vi "DPT RMC Range Calculation.vi"(8 "Error In":errorcluster, 11 "Dryer IMC Data Input":T1={"Measured IMC (lbs)"=7.0, "Actual Initial RMC (%)"=7.0, "RMC (Desired %)"=100.0, "Bone Dry Wt(lbs)"=7.0, "Tolerance(%)"=5.0, "Actual Final RMC (%)"=7.0, "CEF (lbf/kWh)"=0.0, "Minimum Weight (lbf)"=0.0, "Average Weight (lbf)"=0.0, "Maximum Weight (lbf)"=0.0, "Measured IMC In Range?"=FALSE, "Moisture Reduction Factor"=55.5, "Field Use Factor"=1.04, "Empty Dryer Cold Weigth"=0.0, "Energy Standard"=enum."D2-Automatic Dryer", "Weight Cloth (lbs)"=0.0, "Relative Moisture Content (%)"=0.0, "Relative Moisture Content - Avg (%)"=0.0} {"Maximum Weight (lbf)" format="%03_6g"; "Average Weight (lbf)" format="%03_6g"; "Minimum Weight (lbf)" format="%03_6g"; "CEF (lbf/kWh)" format="%03_6g"; "Actual Final RMC (%)" format="%03_6g"; "Tolerance(%)" format="%0#_6g"; "Bone Dry Wt(lbs)" format="%03_6g"; "RMC (Desired %)" format="%0#_6g"; "Actual Initial RMC (%)" format="%03_6g"; "Measured IMC (lbs)" format="%0#_6g"}) -> (0 "Error Out":errorcluster, 3 "Dryer IMC Data Output":T1={"Measured IMC (lbs)"=7.0, "Actual Initial RMC (%)"=7.0, "RMC (Desired %)"=100.0, "Bone Dry Wt(lbs)"=7.0, "Tolerance(%)"=5.0, "Actual Final RMC (%)"=7.0, "CEF (lbf/kWh)"=0.0, "Minimum Weight (lbf)"=0.0, "Average Weight (lbf)"=0.0, "Maximum Weight (lbf)"=0.0, "Measured IMC In Range?"=FALSE, "Moisture Reduction Factor"=55.5, "Field Use Factor"=1.04, "Empty Dryer Cold Weigth"=0.0, "Energy Standard"=enum."D2-Automatic Dryer", "Weight Cloth (lbs)"=0.0, "Relative Moisture Content (%)"=0.0, "Relative Moisture Content - Avg (%)"=0.0} {"Maximum Weight (lbf)" format="%03_6g"; "Average Weight (lbf)" format="%03_6g"; "Minimum Weight (lbf)" format="%03_6g"; "CEF (lbf/kWh)" format="%03_6g"; "Actual Final RMC (%)" format="%03_6g"; "Tolerance(%)" format="%0#_6g"; "Bone Dry Wt(lbs)" format="%03_6g"; "RMC (Desired %)" format="%0#_6g"; "Actual Initial RMC (%)" format="%03_6g"; "Measured IMC (lbs)" format="%0#_6g"})   [LabVIEW 2020, in "File Setup.lvlib"]
uses:
  File Setup.lvlib
  Type Definition/DPT IMC Data.ctl
  Washer DOE/Type Definitions/DOE Dryer Standard.ctl
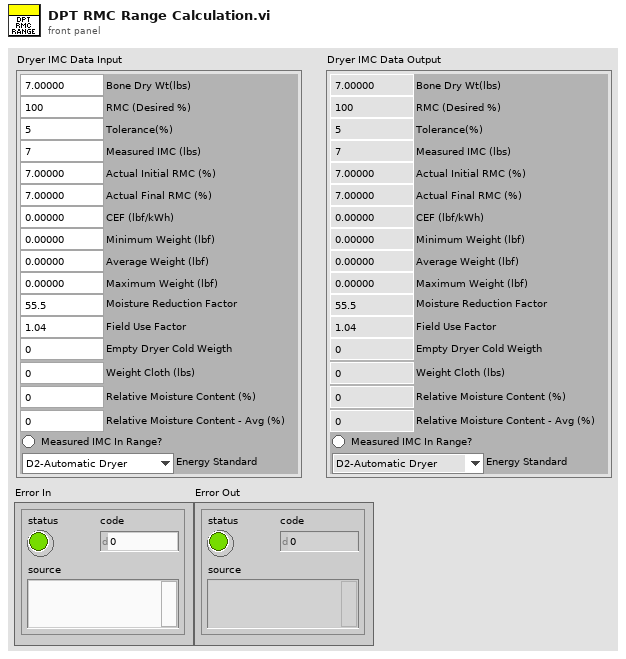
[diagram p1: front panel]
types:
  T1 = typedef "DPT IMC Data.ctl" = cluster{"Measured IMC (lbs)":dbl, "Actual Initial RMC (%)":dbl, "RMC (Desired %)":dbl, "Bone Dry Wt(lbs)":dbl, "Tolerance(%)":dbl, "Actual Final RMC (%)":dbl, "CEF (lbf/kWh)":dbl, "Minimum Weight (lbf)":dbl, "Average Weight (lbf)":dbl, "Maximum Weight (lbf)":dbl, "Measured IMC In Range?":bool, "Moisture Reduction Factor":dbl, "Field Use Factor":dbl, "Empty Dryer Cold Weigth":dbl, "Energy Standard":T2, "Weight Cloth (lbs)":dbl, "Relative Moisture Content (%)":dbl, "Relative Moisture Content - Avg (%)":dbl}
  T2 = typedef "DOE Dryer Standard.ctl" = enum16{"D2-Automatic Dryer", "D2-Timer Dryer", "D1-Automatic Dryer", "D1-Timer Dryer", "Other"}
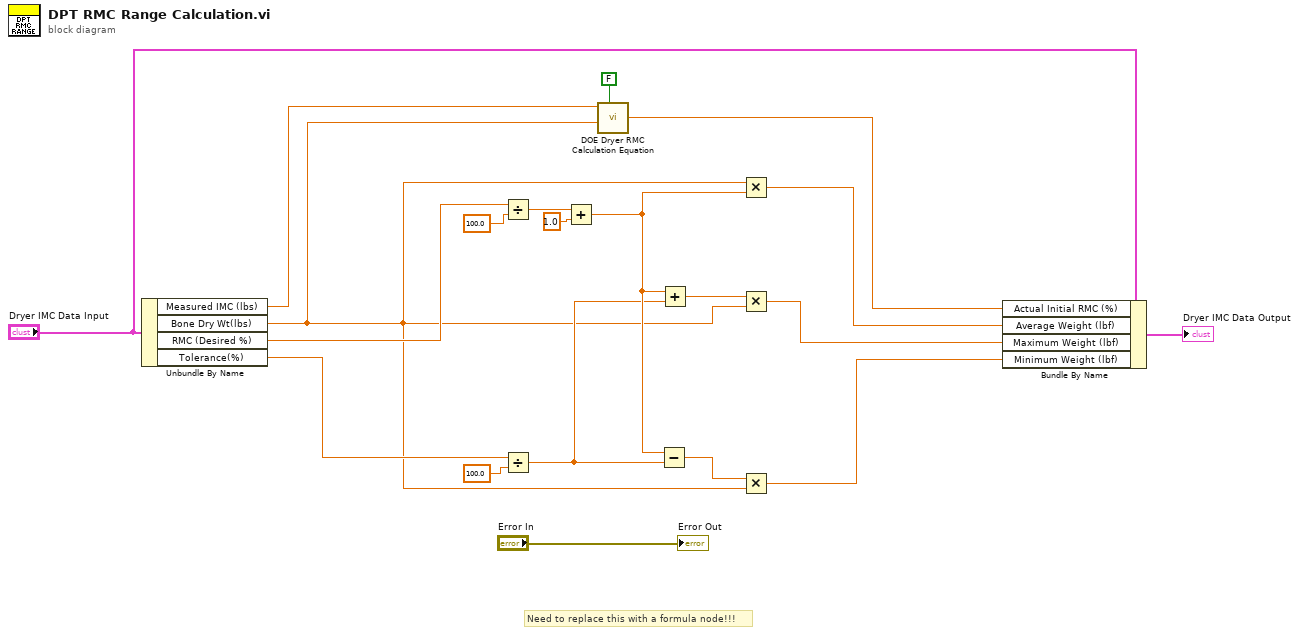
[diagram p0: block diagram]
diagram:
  # "Need to replace this with a formula node!!!"
  n1 = Unbundle By Name("Dryer IMC Data Input") -> ("Measured IMC (lbs)"=w1:dbl, "Bone Dry Wt(lbs)"=w3:dbl, "RMC (Desired %)"=w11:dbl, "Tolerance(%)"=w10:dbl)
  n2 = Divide(x=w11, y=100.0) -> (x/y=w17:dbl)
  n3 = Divide(x=w10, y=100.0) -> (x/y=w13:dbl)
  n4 = Add(x=w17, y=1.0) -> (x+y=w15:dbl)
  n5 = call "DOE Dryer RMC Calculation Equation.vi"("Use Runtime RMC Calculation?"=FALSE, "Bone Dry Weight of Cloth (lbs)"=w3, "Gross Weigth (lbs)"=w1) -> ("Relative Moisture Content (%)"=w2:dbl)  [unwired: 5 in, 3 out]
  n6 = Subtract(x=w15, y=w13) -> (x-y=w19:dbl)
  n7 = Add(x=w15, y=w13) -> (x+y=w18:dbl)
  n8 = Multiply(x=w3, y=w15) -> (x*y=w6:dbl)
  n9 = Multiply(x=w18, y=w3) -> (x*y=w8:dbl)
  n10 = Multiply(x=w19, y=w3) -> (x*y=w7:dbl)
  n11 = Bundle By Name(cluster="Dryer IMC Data Input", "Actual Initial RMC (%)"=w2, "Average Weight (lbf)"=w6, "Maximum Weight (lbf)"=w8, "Minimum Weight (lbf)"=w7) -> (→"Dryer IMC Data Output":T1)
  "Error Out" <- "Error In"
